vi "fix to the line.vi"   [LabVIEW 2018]
uses:
  <vilib>/myRIO/Instrument Drivers/Onboard IO/AI/typedefs/AI Reference.ctl
  <vilib>/myRIO/Common/Instrument Driver Framework/Utilities/typedefs/myRIO Generic Hardware Reference.ctl
  <vilib>/myRIO/Common/Instrument Driver Framework/Utilities/typedefs/Hardware Version Enum.ctl
  <vilib>/myRIO/Common/Instrument Driver Framework/Utilities/typedefs/myRIO v1.0 Reference.ctl
  <vilib>/myRIO/Common/Instrument Driver Framework/Utilities/typedefs/Generic FPGA Reference.ctl
  <vilib>/myRIO/Common/Instrument Driver Framework/myRIO v1.0/AI/typedefs/AI Channels List.ctl
  <vilib>/myRIO/Common/Instrument Driver Framework/myRIO v1.0/AI/typedefs/AI Channels Enum.ctl
  <vilib>/myRIO/Common/Instrument Driver Framework/Utilities/typedefs/Analog Scaling Constants List.ctl
  <vilib>/myRIO/Common/Instrument Driver Framework/Utilities/typedefs/Analog Scaling Constants.ctl
  <vilib>/userdefined/High Color/nirio_resource_hc.ctl
  <vilib>/myRIO/Common/Instrument Driver Framework/Utilities/vis/Is FPGA Ref Available.vi
  <vilib>/myRIO/Common/Instrument Driver Framework/myRIO v1.0/AI/vis/myRIO v1.1 Open AI.vi
  <vilib>/myRIO/Instrument Drivers/Onboard IO/AI/vis/Read.vi
  <vilib>/myRIO/Common/Instrument Driver Framework/Utilities/vis/Validate Channels.vi
  <vilib>/myRIO/Common/Instrument Driver Framework/myRIO v1.0/AI/vis/myRIO v1.0 Reserve AI.vi
  <vilib>/myRIO/Common/Instrument Driver Framework/myRIO v1.0/AI/vis/myRIO v1.0 Build MUX Configuration AI.vi
  <vilib>/myRIO/Common/Instrument Driver Framework/myRIO v1.0/Resource Manager/vis/myRIO v1.0 Reserve Channel List.vi
  <vilib>/myRIO/Common/Instrument Driver Framework/myRIO v1.0/Resource Manager/vis/myRIO v1.0 Reserve Channel.vi
  <vilib>/myRIO/Common/Instrument Driver Framework/myRIO v1.0/Resource Manager/vis/myRIO v1.0 Unreserve Channel.vi
  <vilib>/myRIO/Common/Instrument Driver Framework/myRIO v1.0/Resource Manager/vis/myRIO v1.0 Build Mutex Name.vi
  <vilib>/Utility/VariantDataType/GetNumericInfo.vi
  <vilib>/Utility/error.llb/Error Cluster From Error Code.vi
  <vilib>/myRIO/Common/Instrument Driver Framework/myRIO v1.0/myRIO v1.1 Open.vi
  <vilib>/myRIO/Common/Instrument Driver Framework/myRIO v1.0/AI/vis/myRIO v1.0 Get Scaling Constants AI.vi
  <vilib>/myRIO/Common/Instrument Driver Framework/Utilities/vis/IO Manager.vi
  <vilib>/myRIO/Common/Instrument Driver Framework/Utilities/vis/Configuration Manager.vi
  <vilib>/myRIO/Common/Instrument Driver Framework/myRIO v1.0/myRIO v1.0 Close.vi
  <vilib>/myRIO/Common/Instrument Driver Framework/myRIO v1.0/AI/vis/myRIO v1.0 Read AI.vi
  <vilib>/myRIO/Express VI/Onboard IO/AI/AI Express VI.xnode
  <vilib>/myRIO/Instrument Drivers/Onboard IO/AI/vis/myRIO AI Open.xnode
  <vilib>/myRIO/Instrument Drivers/Onboard IO/AI/AI.lvlib
types:
  T1 = typedef "AI.lvlib/AI Reference.ctl" = cluster{"myRIO Reference":T2, "AI Channels List":T6, "AI Scaling Constants List":T8}
  T2 = typedef "myRIO Generic Hardware Reference.ctl" = cluster{"myRIO Model":T3, "myRIO Hardware Reference":T4}
  T3 = typedef "Hardware Version Enum.ctl" = enum16{"Unknown", "myRIO-1900", "myRIO-1950", "roboRIO", "NI ELVIS RIO CM", "ELVIS III"}
  T4 = typedef "myRIO v1.0 Reference.ctl" = cluster{"Generic FPGA Reference":T5, "Allow multiple opens":bool}
  T5 = typedef "Generic FPGA Reference.ctl" = refnum<k20>
  T6 = typedef "AI Channels List.ctl" = T7[]
  T7 = typedef "AI Channels Enum.ctl" = enum16{"Not Connected", "AudioIn/Left", "AudioIn/Right", "C/AI0", "C/AI1", "A/AI0", "A/AI1", "A/AI2", "A/AI3", "A/AI4", "A/AI5", "A/AI6", "A/AI7", "B/AI0", "B/AI1", "B/AI2", "B/AI3", "B/AI4", "B/AI5", "B/AI6", "B/AI7", "AI/AI0", "AI/AI1", "AI/AI2", "AI/AI3", "A/AI0 (DIFF)", "A/AI1 (DIFF)", "A/AI2 (DIFF)", "A/AI3 (DIFF)", "B/AI0 (DIFF)", "B/AI1 (DIFF)", "B/AI2 (DIFF)", "B/AI3 (DIFF)"}
  T8 = typedef "Analog Scaling Constants List.ctl" = T9[]
  T9 = typedef "Analog Scaling Constants.ctl" = cluster{"LSB Weight (Volts)":dbl, "Offset (Volts)":dbl, "Signed?":bool}
  T10 = typedef "nirio_resource_hc.ctl" = tag
  T11 = enum16{"forward", "backward", "left", "right", "rotate left", "rotate right"}
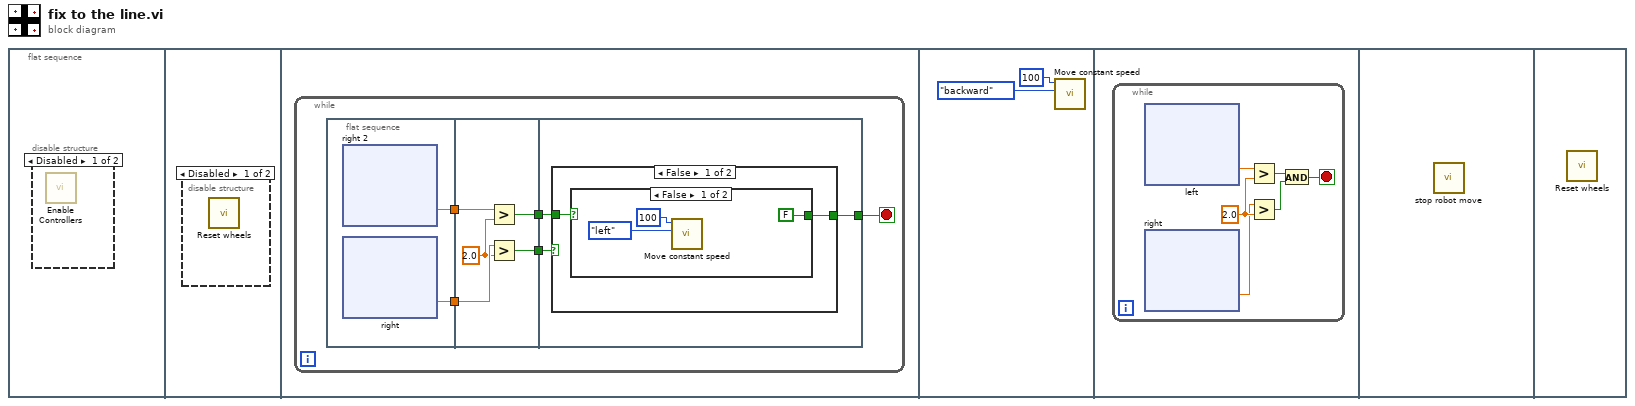
[diagram p0: block diagram]
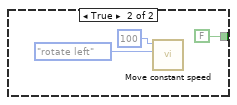
[diagram p4: hidden frame]
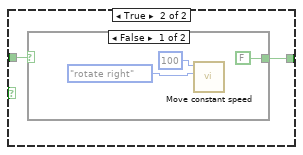
[diagram p5: hidden frame]
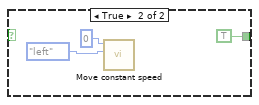
[diagram p6: hidden frame]
diagram:
  n1 = flat-sequence {
    frame #0 {
      n2 = disable-structure shown="Disabled" {
        frame Disabled {
          n3 = call "Enable Controllers.vi"() -> ()  [unwired: 12 in]
        }
        frame Enabled {
        }
      }
    }
    frame #1 {
      n4 = disable-structure shown="Disabled" {
        frame Disabled {
          n5 = call "Reset wheels.vi"() -> ()  [unwired: 12 in]
        }
        frame Enabled {
        }
      }
    }
    frame #2 {
      n6 = while {
        stop <- w1 stop-if-true
        n7 = flat-sequence {
          tunnel: [w7] -> w5
          tunnel: [w6] -> w4
          tunnel: w5 -> [w86]
          tunnel: w4 -> [w85]
          tunnel: [w83] -> w3
          tunnel: [w82] -> w2
          tunnel: w3 -> [w89]
          tunnel: w2 -> [w88]
          tunnel: [w87] -> w1
          frame #0 {
            n8 = xnode "right 2"() -> ("A/AI3 (Pin 9)"=w6:dbl)  [unwired: 1 in, 1 out]
            n9 = xnode "right"() -> ("A/AI0 (Pin 3)"=w7:dbl)  [unwired: 1 in, 1 out]
          }
          frame #1 {
            w84 = 2.0 ("y")
            n10 = Greater?(x=w85, y=w84) -> (0:w82:bool)
            n11 = Greater?(x=w86, y=w84) -> (0:w83:bool)
          }
          frame #2 {
            n12 = case shown="False" w89 {
              tunnel: w88 -> [w91 w99]
              tunnel: [w90 w98] -> w87
              frame False {
                n13 = case shown="False" w91 {
                  tunnel: [FALSE FALSE] -> w90
                  frame False {
                    n14 = call "Move constant speed.vi"("Enum"=T11."left", "speed"=100) -> ()  [unwired: 10 in]
                  }
                  frame True {
                    n15 = call "Move constant speed.vi"("Enum"=T11."rotate left", "speed"=100) -> ()  [unwired: 10 in]
                  }
                }
              }
              frame True {
                n16 = case shown="False" w99 {
                  tunnel: [FALSE TRUE] -> w98
                  frame False {
                    n17 = call "Move constant speed.vi"("Enum"=T11."rotate right", "speed"=100) -> ()  [unwired: 10 in]
                  }
                  frame True {
                    n18 = call "Move constant speed.vi"("Enum"=T11."left", "speed"=0) -> ()  [unwired: 10 in]
                  }
                }
              }
            }
          }
        }
      }
    }
    frame #3 {
      n19 = call "Move constant speed.vi"("Enum"=T11."backward", "speed"=100) -> ()  [unwired: 10 in]
    }
    frame #4 {
      n20 = while {
        stop <- w108 stop-if-true
        w113 = 2.0 ("y")
        n21 = xnode "left"() -> ("A/AI1 (Pin 5)"=w112:dbl)  [unwired: 1 in, 1 out]
        n22 = xnode "right"() -> ("A/AI0 (Pin 3)"=w111:dbl)  [unwired: 1 in, 1 out]
        n23 = Greater?(x=w112, y=w113) -> (0:w110:bool)
        n24 = Greater?(x=w111, y=w113) -> (0:w109:bool)
        n25 = And(x=w110, y=w109) -> (x .and. y?=w108:bool)
      }
    }
    frame #5 {
      n26 = call "stop robot move.vi"() -> ()  [unwired: 12 in]
    }
    frame #6 {
      n27 = call "Reset wheels.vi"() -> ()  [unwired: 12 in]
    }
  }
